vi "ROIAutoSearch.vi"(0 "multi image in":i32[][](array[numeric]), 1 "Correlation \nTreshold\n(0..1)":dbl=0.6, 2 "Proximity (ROI size units)":dbl=0.45, 5 "Autofind?":bool, 7 "ROI (pix)":i32=60 min=0 step=2, 9 "template image in":u8[][](array[numeric]), 11 "ROI array in":u32[][](array[numeric]), 12 "error out":errorcluster) -> (4 "Reg of Int of the bead 2":u8[][](graph), 6 "ROI array out":u32[][](array[numeric]), 15 "error out 3":errorcluster)   [LabVIEW 2011, in "OfflineTracker.lvlib"]
doc: "This vi uses a pre-chosen single bead image to find the closest resembling sub-images in a larger image containing multiple beads. Output is the corresponding ROI list. JacobKers09"
uses:
  OfflineTracker.lvlib
panel:
  out "Sorted array":dbl[][](array[numeric])
  out "size(s)":i32[](array[numeric])
  out "Best centers":dbl[][](array[numeric])
  out "ori image 4":dbl[][](graph)
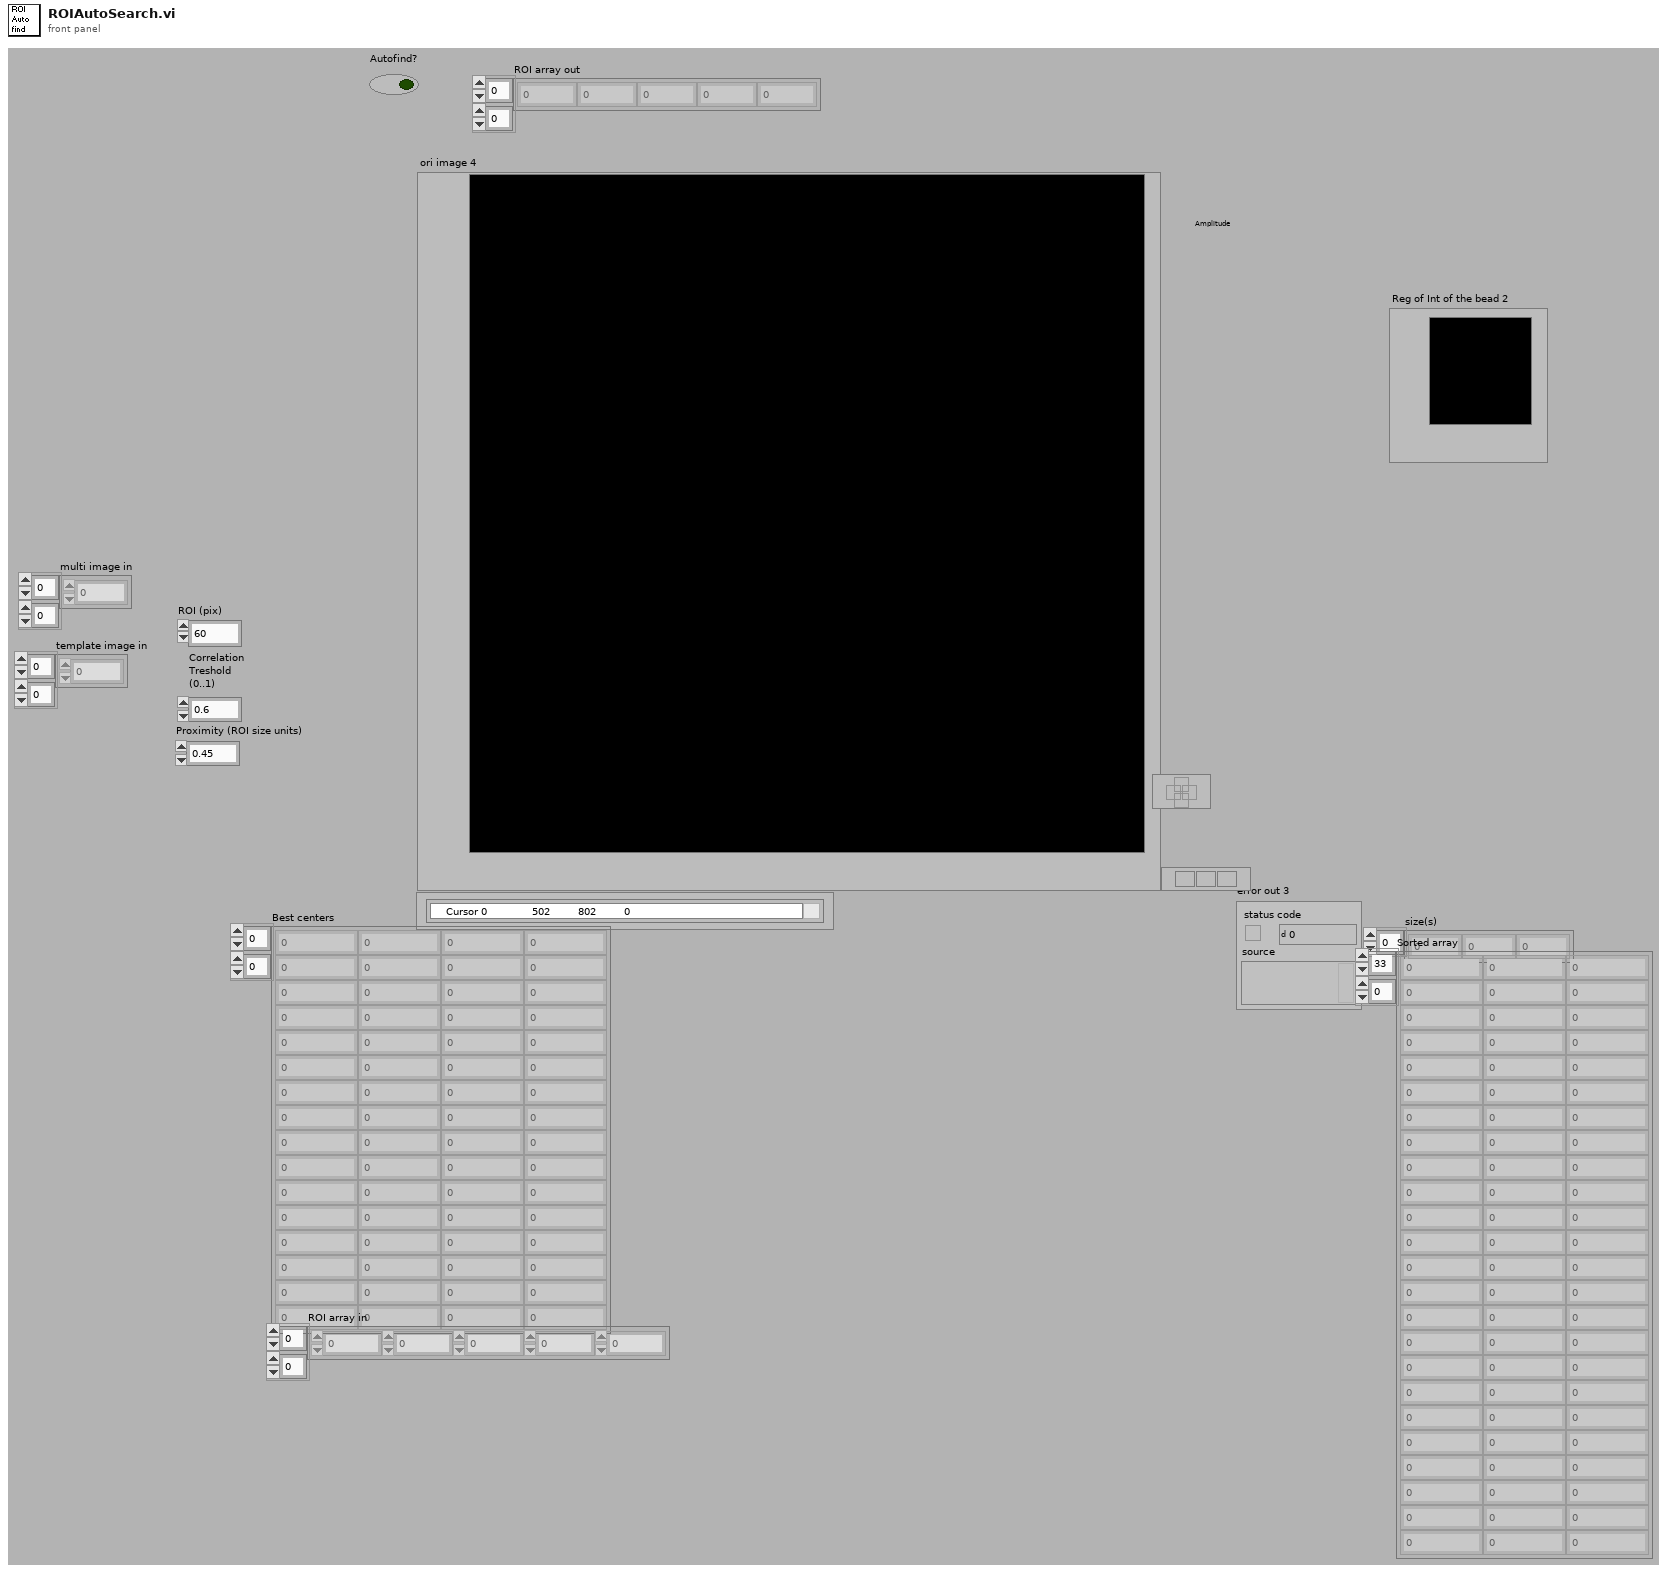
[diagram p1: front panel]
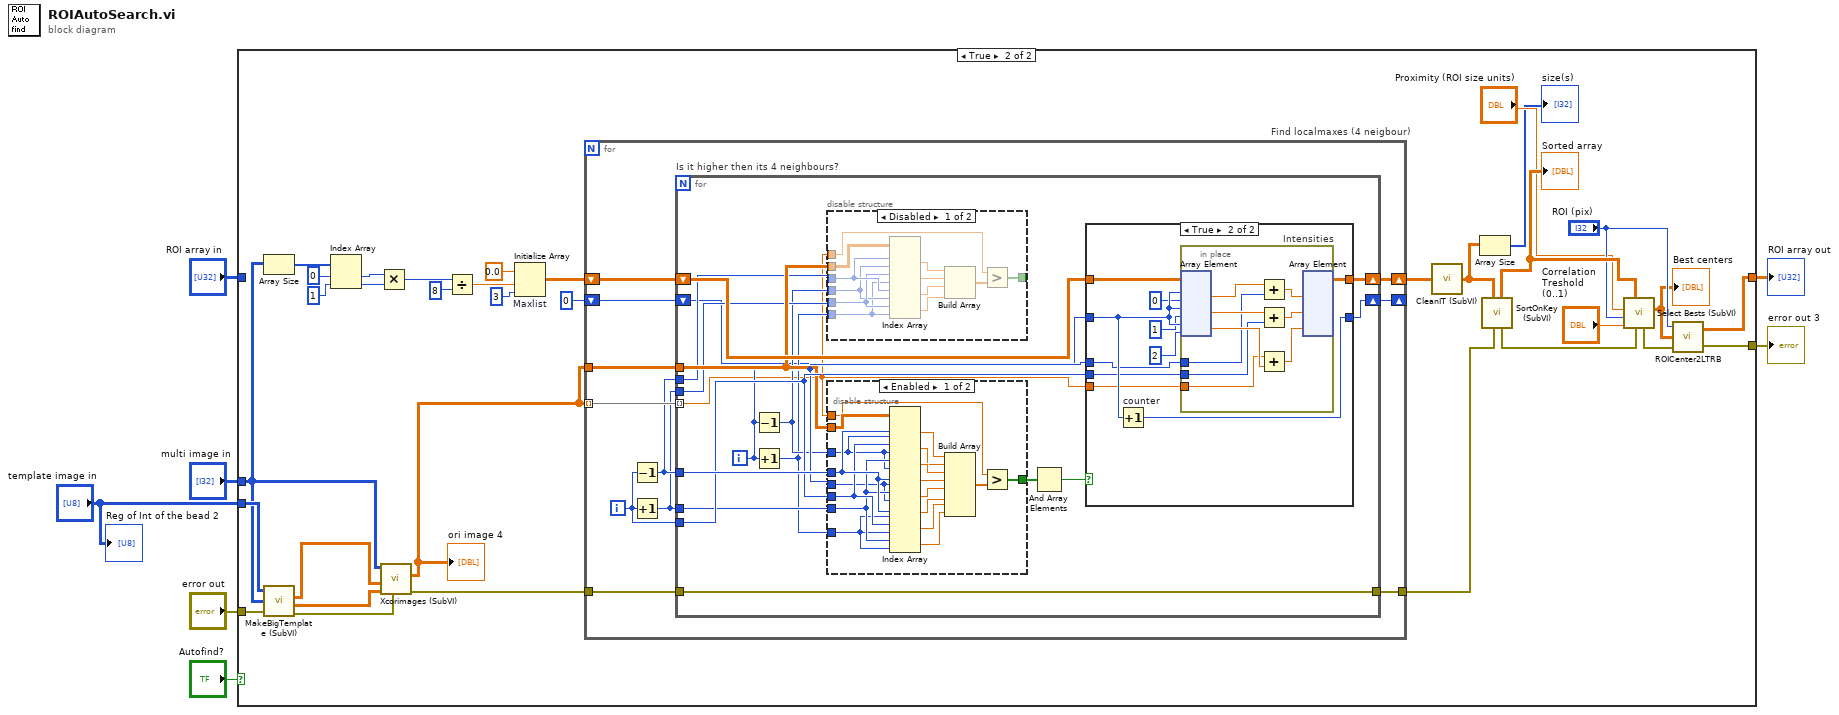
[diagram p0: block diagram]
diagram:
  n1 = case shown="True" "Autofind?" {
    tunnel: "error out" -> [w9 w27]
    tunnel: [w9 w25] -> w6
    tunnel: [w8 w31] -> w5
    tunnel: "template image in" -> [_ w26]
    tunnel: "ROI array in" -> [w8 _]
    tunnel: "multi image in" -> [_ w19]
    frame False {
    }
    frame True {
      n2 = Array Size(array=w19) -> (size(s)=w18:i32[])
      n3 = call "MakeBigTemplate (SubVI).vi"("template image in"=w26, "multi image in"=w19, "error out"=w27) -> ("template pic"=w22:dbl[][], "smooth template, normalized"=w21:dbl[][], "error out 2"=w34:errorcluster)  [unwired: 1 in]
      n4 = Index Array(array=w18, index #1=0 ("index"), index #2=1 ("index")) -> (element #1=w15:i32, element #2=w14:i32)
      n5 = Multiply(x=w15, y=w14) -> (x*y=w13:i32)
      n6 = call "Xcorimages (SubVI).vi"("error out"=w34, "ROI smooth template in"=w21, "Bead template in"=w22, "multi image in"=w19) -> ("error out 2"=w33:errorcluster, "Array"=w39:dbl[][])  [unwired: 5 out]
      "ori image 4" <- w39
      n7 = Divide(x=w13, y=8) -> (x/y=w11:dbl)
      n8 = Initialize Array "Maxlist"(0.0 ("element"), w11, 3 ("dimension size")) -> (w40:dbl[][])
      n9 = for "Find localmaxes (4 neigbour)" {
        tunnel: w39 -> [w53] mode=indexing
        tunnel: w39 -> [w50]
        shift-right: [w51] -> w24
        shift-left: w40 -> [w52]
        tunnel: w33 -> [w49]
        tunnel: [w48] -> w38
        shift-right: [w44] -> _
        shift-left: u32 0 ("element") -> [w43]
        i -> [w47]
        n10 = Decrement(x=w47) -> (x-1=w46:i32)
        n11 = Increment(x=w47) -> (x+1=w45:i32)
        n12 = for "Is it higher then its 4 neighbours?" {
          tunnel: w53 -> [w57] mode=indexing
          tunnel: w47 -> [w65]
          tunnel: w50 -> [w63]
          shift-right: [w69] -> w51
          shift-left: w52 -> [w70]
          tunnel: w49 -> [w68]
          tunnel: [w68] -> w48
          tunnel: w46 -> [w66]
          tunnel: w45 -> [w64]
          tunnel: w46 -> [w61]
          tunnel: w45 -> [w60]
          shift-right: [w54] -> w44
          shift-left: w43 -> [w55]
          i -> [w62]
          n13 = Decrement(x=w62) -> (x-1=w59:i32)
          n14 = Increment(x=w62) -> (x+1=w58:i32)
          n15 = disable-structure shown="Disabled" {
            disable-tunnel: w63 -> [w82 _]
            disable-tunnel: w61 -> [w81 _]
            disable-tunnel: w60 -> [w80 _]
            disable-tunnel: w59 -> [w79 _]
            disable-tunnel: w58 -> [w78 _]
            disable-tunnel: w57 -> [w73 _]
            disable-tunnel: [w71 _] -> _
            frame Disabled {
              n16 = Index Array(array=w82, index (row) #1=w81, index (col) #1=w79, index (row) #2=w80, index (col) #2=w78, index (row) #3=w81, index (col) #3=w79, index (row) #4=w80, index (col) #4=w78) -> (element #1=w77:dbl, element #2=w76:dbl, element #3=w75:dbl, element #4=w74:dbl)
              n17 = Build Array(w77, w76, w75, w74) -> (w72:dbl[])
              n18 = Greater?(x=w73, y=w72) -> (0:w71:bool[])
            }
            frame Enabled {
            }
          }
          n19 = disable-structure shown="Enabled" {
            disable-tunnel: w66 -> [w91 _]
            disable-tunnel: w65 -> [w90 _]
            disable-tunnel: w64 -> [w89 _]
            disable-tunnel: w63 -> [w88 _]
            disable-tunnel: w62 -> [w87 _]
            disable-tunnel: w59 -> [w86 _]
            disable-tunnel: w58 -> [w85 _]
            disable-tunnel: w57 -> [w84 _]
            disable-tunnel: [w83 _] -> w56
            frame Enabled {
              n20 = Index Array(array=w88, index (row) #1=w91, index (col) #1=w86, index (row) #2=w90, index (col) #2=w86, index (row) #3=w89, index (col) #3=w86, index (row) #4=w91, index (col) #4=w87, index (row) #5=w89, index (col) #5=w87, index (row) #6=w91, index (col) #6=w85, index (row) #7=w90, index (col) #7=w85, index (row) #8=w89, index (col) #8=w85) -> (element #1=w92:dbl, element #2=w93:dbl, element #3=w94:dbl, element #4=w95:dbl, element #5=w97:dbl, element #6=w98:dbl, element #7=w99:dbl, element #8=w100:dbl)
              n21 = Build Array(w92, w93, w94, w95, w97, w98, w99, w100) -> (w96:dbl[])
              n22 = Greater?(x=w84, y=w96) -> (0:w83:bool[])
            }
            frame Disabled {
            }
          }
          n23 = And Array Elements(Boolean array=w56) -> (logical AND=w67:bool)
          n24 = case shown="True" w67 {
            tunnel: w70 -> [w102 w111]
            tunnel: w57 -> [_ w103]
            tunnel: w65 -> [_ w104]
            tunnel: w62 -> [_ w105]
            tunnel: [w102 w106] -> w69
            tunnel: w55 -> [w101 w110]
            tunnel: [w101 w112] -> w54
            frame False {
            }
            frame True {
              n25 = Increment "counter"(x=w110) -> (x+1=w112:u32)
              n26 = in-place "Intensities" {
                in-place-border: w105 -> [w115]
                in-place-border: w104 -> [w114]
                in-place-border: w103 -> [w113]
                n27 = in-place-array #1(w111, w110, 0, w110, 1, w110, 2) -> (w121:dbl, w120:dbl, w119:dbl)
                n28 = Add(x=w121, y=w115) -> (x+y=w118:dbl)
                n29 = Add(x=w120, y=w114) -> (x+y=w117:dbl)
                n30 = Add(x=w113, y=w119) -> (x+y=w116:dbl)
                n31 = in-place-array #1(w118, w117, w116) -> (w106:dbl[][])  [unwired: 6 out]
              }
            }
          }
        }
      }
      n32 = call "CleanIT (SubVI).vi"("in array"=w24) -> ("pre-cleaned Array"=w20:dbl[][])
      n33 = Array Size(array=w20) -> (size(s)=→"size(s)":i32[])
      n34 = call "SortOnKey (SubVI).vi"("error out"=w38, "Unsorted Array"=w20) -> ("error out 2"=w36:errorcluster, "Sorted array"=w37:dbl[][])  [unwired: 2 in, 6 out]
      "Sorted array" <- w37
      n35 = call "Select Bests (SubVI).vi"("error out 3"=w36, "Candidate beads"=w37, "CorrelationTreshold"="Correlation \nTreshold\n(0..1)", "Roi size"="ROI (pix)", "Proximity (ROI size units)"="Proximity (ROI size units)") -> ("Good Beads"=w29:dbl[][], "error out 2"=w32:errorcluster)  [unwired: 1 in, 4 out]
      "Best centers" <- w29
      n36 = call "ROICenter2LTRB.vi"("error out 3"=w32, "Selected array"=w29, "ROI (pix)"="ROI (pix)") -> ("error out 2"=w25:errorcluster, "Array"=w31:dbl[][])
    }
  }
  "error out 3" <- w6
  "ROI array out" <- w5
  "Reg of Int of the bead 2" <- "template image in"
